vi "Triggered Sync.vi"(8 "error in":errorcluster, 11 "4300 in":refnum<class "4300.lvclass">) -> (0 "error out":errorcluster, 3 "4300 out":refnum<class "4300.lvclass">)   [LabVIEW 2019, in "4300.lvlib" / "4300.lvclass"]
uses:
  Library/4300.lvclass
  C:/Users/Public/Documents/Development/builds/Instruments/AnalogInput.lvlibp/Library/AnalogInput.lvclass
  Library/4300.lvclass/4300.ctl
  builds/Instruments/AnalogInput.lvlibp/Accessors/Triggering/Read Trigger Settings.vi
  <vilib>/DAQmx/configure/timing.llb/DAQmx Timing (Sample Clock).vi
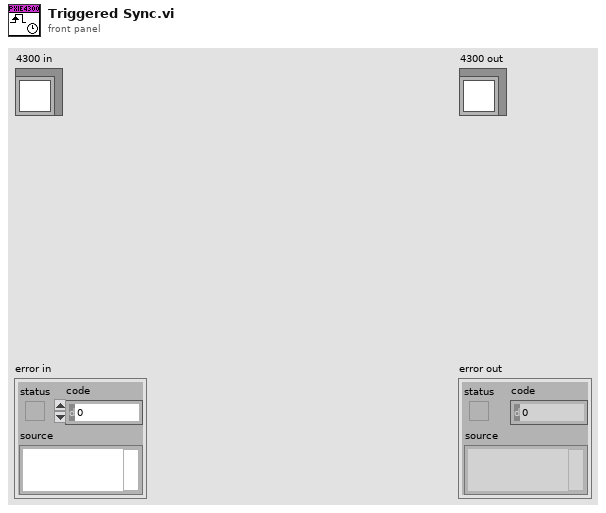
[diagram p1: front panel]
types:
  T1 = typedef "AnalogInput.lvlibp/AnalogInput.lvclass/User Trigger Settings.ctl" = cluster{"Timeout":dbl, "Level":dbl, "Slope":T2, "samples per channel":i32, "Sample Rate (10k)":dbl, "pretrigger samples":u32}
  T2 = typedef "AnalogInput.lvlibp/AnalogInput.lvclass/Trigger_Slope.ctl" = enum16{"Rising", "Falling"}
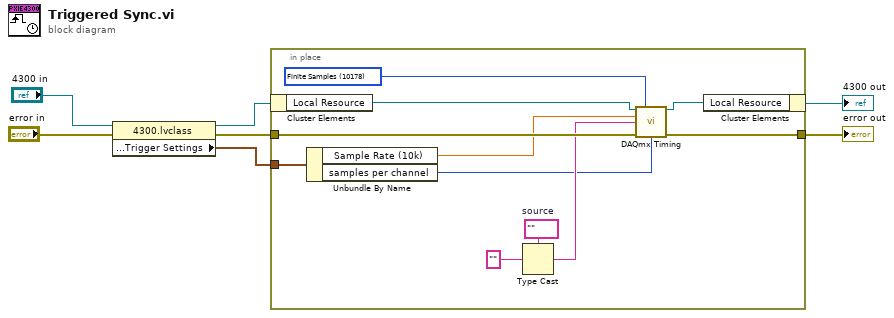
[diagram p0: block diagram]
diagram:
  n1 = property class="4300.lvclass"(reference="4300 in", error in="error in") -> (reference out=w2:refnum<class "4300.lvclass">, error out=w7:errorcluster, "Accessors:Triggering:Trigger Settings"=w5:T1)
  n2 = in-place {
    in-place-border: w7 -> [w18]
    in-place-border: [w17] -> w6
    in-place-border: w5 -> [w13]
    w11 = 10178 items=["Finite Samples"=10178, "Continuous Samples"=10123, "Hardware Timed Single Point"=12522] ("sample mode")
    w16 = tag ""  # source
    n3 = in-place-cluster #1(w2) -> ("Local Resource"=w10:refnum<k21>)
    n4 = Unbundle By Name(w13) -> ("Sample Rate (10k)"=w8:dbl, "samples per channel"=w14:i32)
    n5 = Type Cast(type=w16, x="" ("Trig Source")) -> (*(type *) &x=w15:tag)
    n6 = call-poly <vilib>:"DAQmx Timing.vi"("task/channels in"=w10, "sample mode"=w11, "samples per channel"=w14, "rate"=w8, "source"=w15, "error in"=w18) -> ("task out"=w9:refnum<k21>, "error out"=w17:errorcluster)  [unwired: 8 in]
    n7 = in-place-cluster #1("Local Resource"=w9) -> (→"4300 out":refnum<class "4300.lvclass">)
  }
  "error out" <- w6
